vi "funcaoAvaliacaoGoleiroBolaPertoArea.vi"(8 "balls":T1[](array[typedef]), 9 "Robot in":T2, 10 "Estado_Atual":T7(ring), 11 "IA State":T8={"our_robots"=[], "enemy_robots"=[], "balls"=[], "geometry"={"field_length"=0, "field_width"=0, "goal_width"=0, "goal_depth"=0, "center_circle_radius"=0, "defense_width"=0, "defense_depth"=0, "free_kick_from_defense_dist"=0, "penalty_spot_from_field_line_dist"=0, "penalty_line_from_spot_dist"=0, "half_moon_depth"=0, "half_moon_width"=0}, "IA Judge"={"stage"="", "command"="", "our_goalie_id"=0.0, "enemy_goalie_id"=0.0, "command enum"=enum."Halt", "Time"=enum."Azul"}, "Received Timestamp"=timestamp(0 s since 1904-01-01), "Events"={"Touch"=FALSE, "id touch"=0.0, "Ball out of \nVision"=FALSE, "Ball inside \nGoalie area"=FALSE, "Robot not responding"=FALSE, "Robots responding status"=[1.0, 1.0, 1.0, 1.0, 1.0, 1.0], "Enemy Ball \nPossession"=FALSE, "Id ini Possession"=0.0, "Ball Possesion"=FALSE, "Id Possesion"=0.0, "Ball at\nour goal side"=FALSE, "Ball at\ntouchline"=FALSE, "Ball at\nenemy goal side"=FALSE}}) -> (3 "Estado_Novo":T7(ring))   [LabVIEW 2018]
uses:
  2019/VSS/Core/AI Input.ctl
  2019/VSS/Core/AI Robot.ctl
  2019/VSS/Intel/Functions Enum.ctl
  2019/VSS/Intel/AttackerStates.ctl
  2019/VSS/Path Planning/RRT/PathDests.ctl
  2019/VSS/Path Planning/RRT/PathDest.ctl
  2019/VSS/Core/AI Ball.ctl
  2019/VSS/Core/Field Size.ctl
  2019/VSS/Core/AI Judge.ctl
  2019/VSS/Intel/Command Enum.ctl
  2019/VSS/Util/Events/Events.ctl
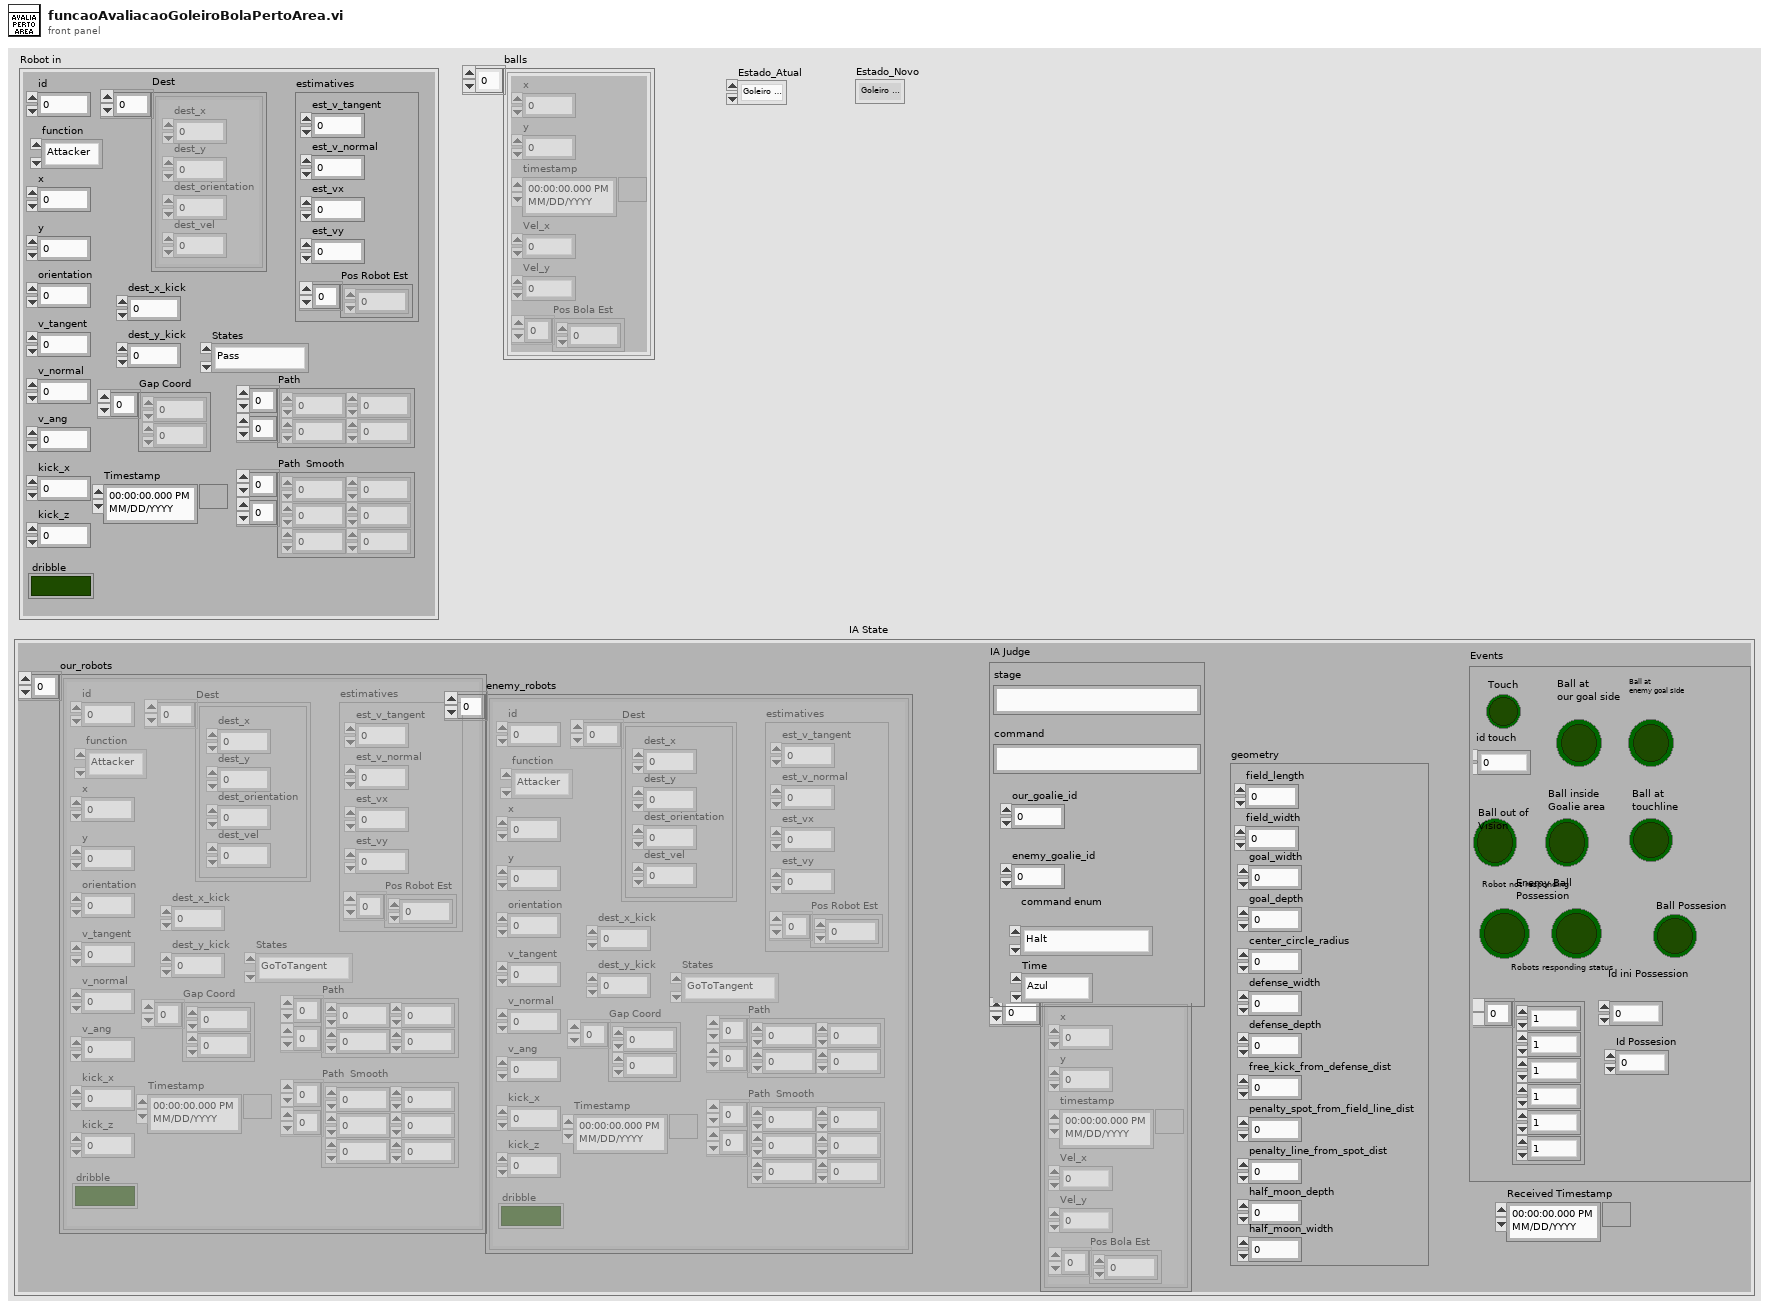
[diagram p1: front panel]
types:
  T1 = typedef "AI Ball.ctl" = cluster{"x":dbl, "y":dbl, "timestamp":timestamp, "Vel_x":dbl, "Vel_y":dbl, "Pos Bola Est":dbl[]}
  T2 = typedef "AI Robot.ctl" = cluster{"id":u32, "function":T3, "x":dbl, "y":dbl, "orientation":dbl, "v_tangent":dbl, "v_normal":dbl, "v_ang":dbl, "kick_x":dbl, "kick_z":dbl, "dribble":bool, "Timestamp":timestamp, "estimatives":cluster{"est_v_tangent":dbl, "est_v_normal":dbl, "est_vx":dbl, "est_vy":dbl, "Pos Robot Est":dbl[]}, "dest_x_kick":dbl, "dest_y_kick":dbl, "Gap Coord":dbl[], "States":T4, "Path ":dbl[][], "Path  Smooth":dbl[][], "Dest":T5}
  T3 = typedef "Functions Enum.ctl" = enum16{"Attacker", "Goalie", "Defender", "Striker", "Goto 0", "Dummy", "Kicker", "ZigZag"}
  T4 = typedef "AttackerStates.ctl" = enum16{"Pass", "GoToTangent", "BallGetting", "GoToKick", "Rotate anti-clockwise", "Rotate Clockwise", ""}
  T5 = typedef "PathDests.ctl" = T6[]
  T6 = typedef "PathDest.ctl" = cluster{"dest_x":dbl, "dest_y":dbl, "dest_orientation":dbl, "dest_vel":dbl}
  T7 = enum16{"Goleiro fora da área", "Alinhar com a bola", "Alinhar com a trave", "Rotacionar", "Aproximar-se da bola", "Posicionar-se na frente da bola"}
  T8 = typedef "AI Input.ctl" = cluster{"our_robots":T2[], "enemy_robots":T2[], "balls":T1[], "geometry":T9, "IA Judge":T10, "Received Timestamp":timestamp, "Events":T12}
  T9 = typedef "Field Size.ctl" = cluster{"field_length":u32, "field_width":u32, "goal_width":u32, "goal_depth":u32, "center_circle_radius":u32, "defense_width":u32, "defense_depth":u32, "free_kick_from_defense_dist":u32, "penalty_spot_from_field_line_dist":u32, "penalty_line_from_spot_dist":u32, "half_moon_depth":u32, "half_moon_width":u32}
  T10 = typedef "AI Judge.ctl" = cluster{"stage":string, "command":string, "our_goalie_id":dbl, "enemy_goalie_id":dbl, "command enum":T11, "Time":enum16{"Azul", "Amarelo"}}
  T11 = typedef "Command Enum.ctl" = enum16{"Halt", "Stop", "Force Start", "PKA Normal Start", "Prepare Kickoff Ally", "PKE Normal Start", "Prepare Kickoff Enemy", "Prepare Penalty Ally", "PPA Normal Start", "Prepare Penalty Enemy", "PPE Normal Start", "Ball Placement Enemy Up", "Ball Placement Enemy Down", "Ball Placement Ally Up", "Ball Placement Ally Mid", "Ball Placement Ally Down", "Indirect Free Enemy", "Indirect Free Ally", "Timeout Enemy", "Timeout Ally", "Goal Enemy", "Goal Ally", "Normal Half Time", "Extra Time Break", "Extra Half Time", "None", "Post Game"}
  T12 = typedef "Events.ctl" = cluster{"Touch":bool, "id touch":dbl, "Ball out of \nVision":bool, "Ball inside \nGoalie area":bool, "Robot not responding":bool, "Robots responding status":dbl[], "Enemy Ball \nPossession":bool, "Id ini Possession":dbl, "Ball Possesion":bool, "Id Possesion":dbl, "Ball at\nour goal side":bool, "Ball at\ntouchline":bool, "Ball at\nenemy goal side":bool}
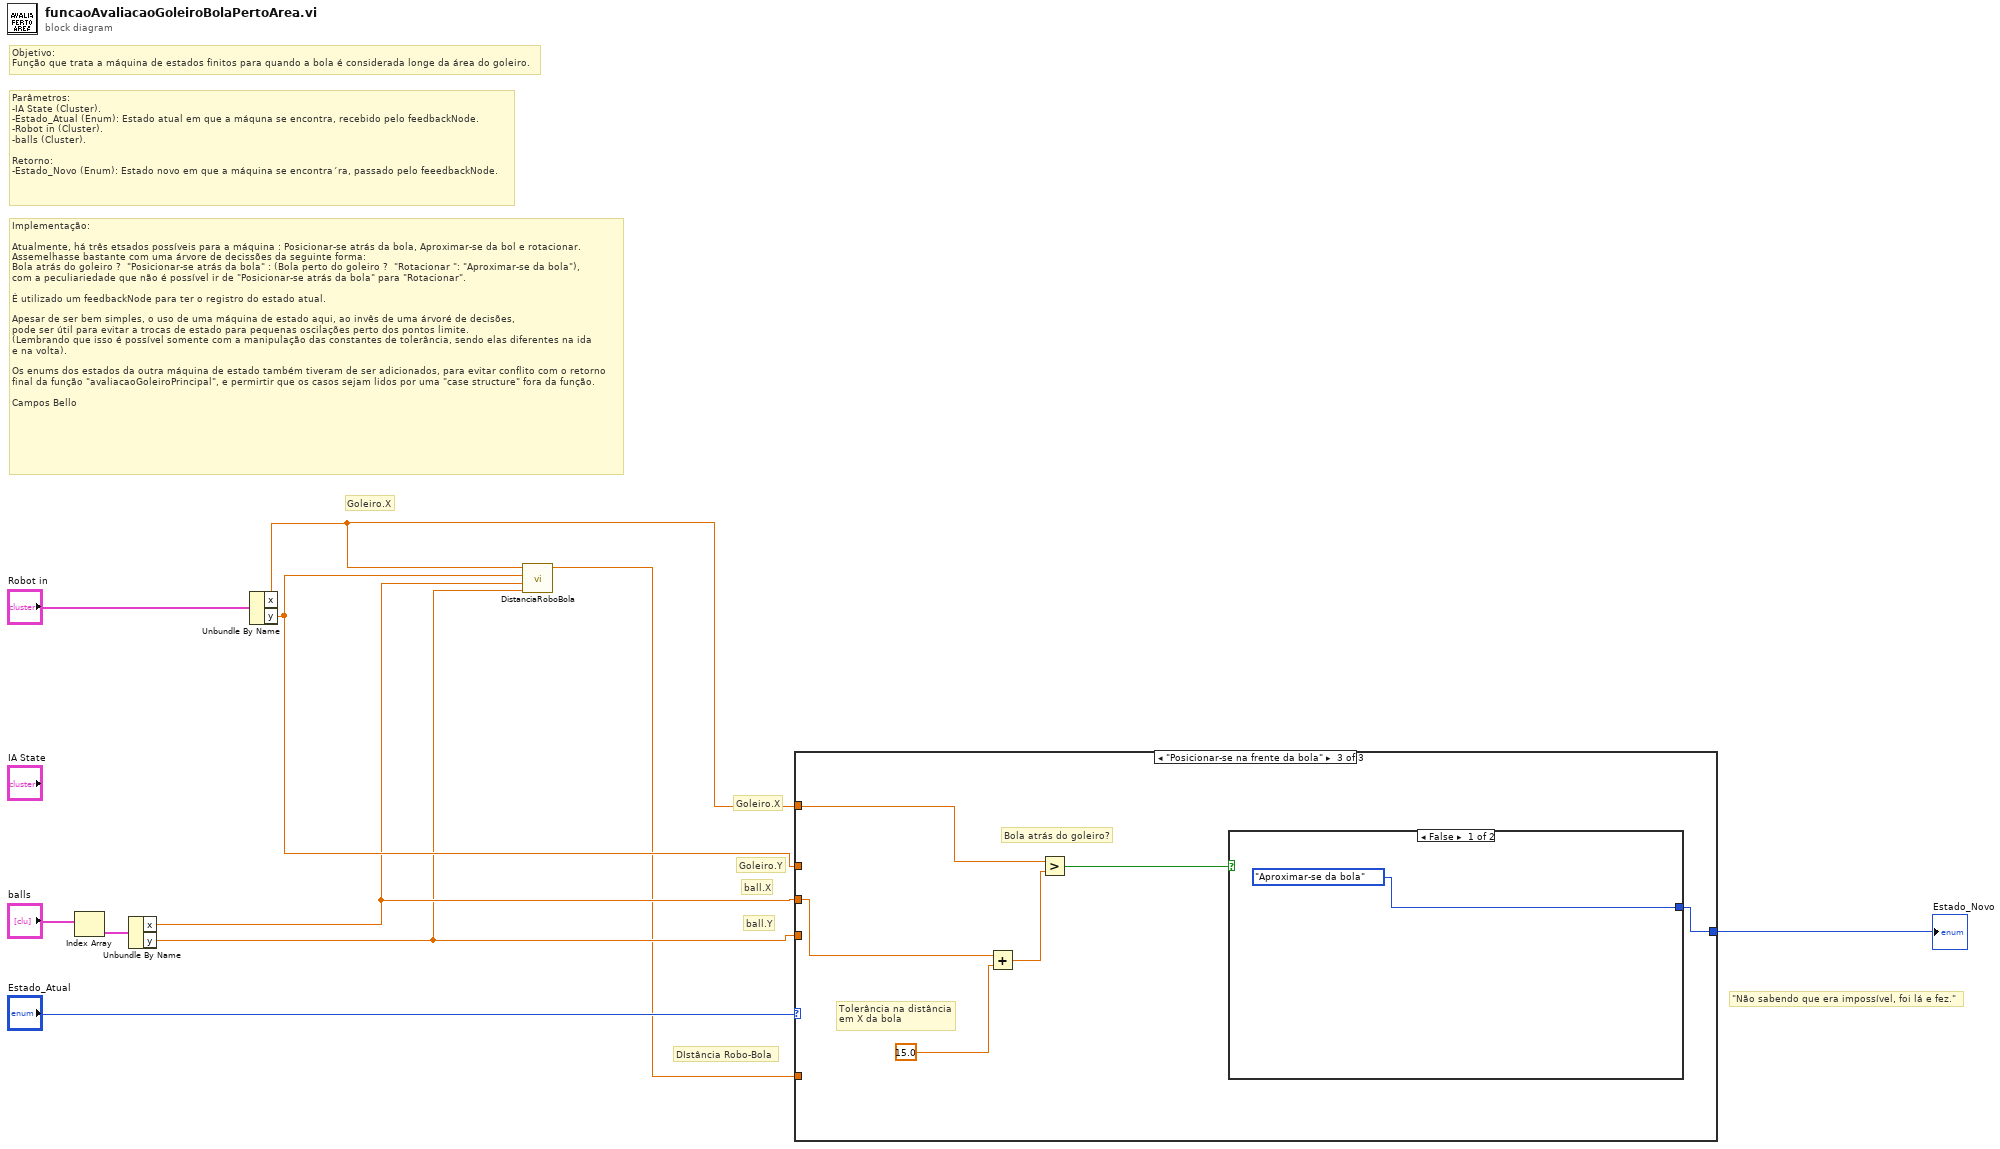
[diagram p0: block diagram]
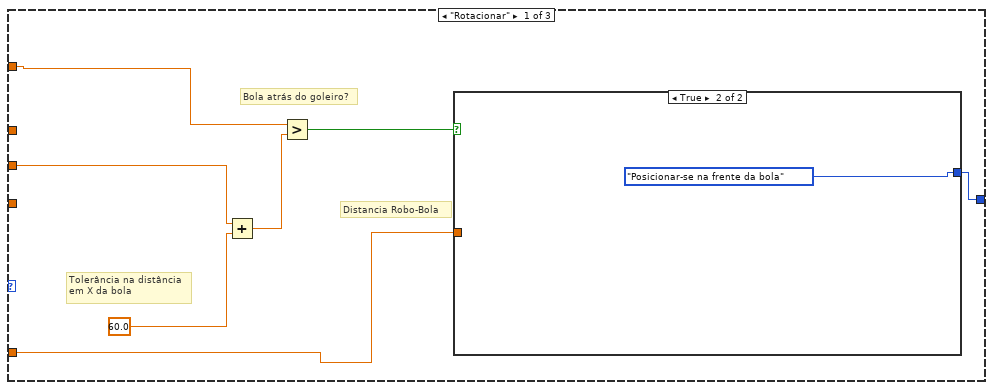
[diagram p2: hidden frame]
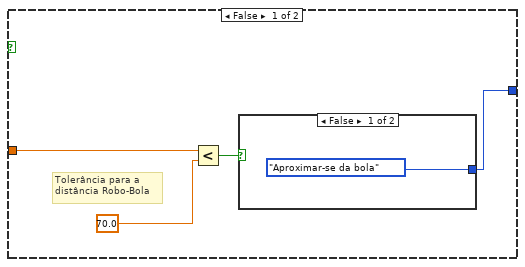
[diagram p3: hidden frame]
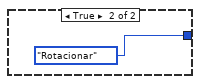
[diagram p4: hidden frame]
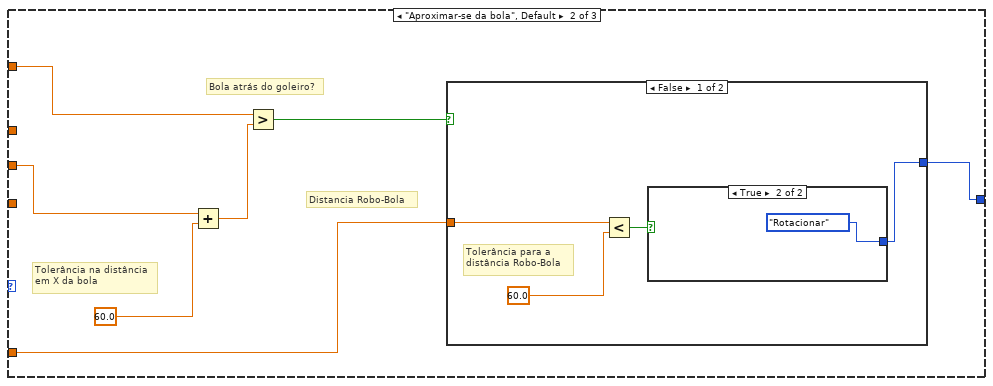
[diagram p5: hidden frame]
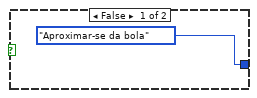
[diagram p6: hidden frame]
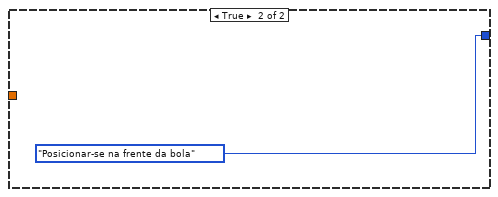
[diagram p7: hidden frame]
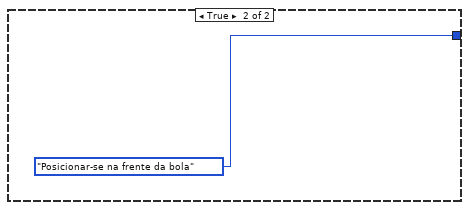
[diagram p8: hidden frame]
diagram:
  # "\"Não sabendo que era impossível, foi lá e fez.\""
  # "Implementação:\n\nAtualmente, há três etsados possíveis para a máquina : Posicionar-se atrás da bola, Aproximar-se da bol e rotacionar.\nAssemelhasse bastante com uma árvore de decissões da seguinte forma: \nBola atrás do goleiro ?  \"Posicionar-se atrás da bola\" : (Bola perto do goleiro ?  \"Rotacionar \": \"Aproximar-se da bola\"), \ncom a peculiariedade que não é possível ir de \"Posicionar-se atrás da bola\" para \"Rotacionar\".\n\nÉ utilizado um feedbackNode para ter o registro do estado atual.\n\nApesar de ser bem simples, o uso de uma máquina de estado aqui, ao invês de uma árvoré de decisões, \npode ser útil para evitar a trocas de estado para pequenas oscilações perto dos pontos limite.\n(Lembrando que isso é possível somente com a manipulação das constantes de tolerância, sendo elas diferentes na ida \ne na volta).\n\nOs enums dos estados da outra máquina de estado também tiveram de ser adicionados, para evitar conflito com o retorno\nfinal da função \"avaliacaoGoleiroPrincipal\", e permirtir que os casos sejam lidos por uma \"case structure\" fora da função.\n\nCampos Bello"
  # "Parâmetros:\n-IA State (Cluster).\n-Estado_Atual (Enum): Estado atual em que a máquna se encontra, recebido pelo feedbackNode.\n-Robot in (Cluster).\n-balls (Cluster).\n\nRetorno:\n-Estado_Novo (Enum): Estado novo em que a máquina se encontra´ra, passado pelo feeedbackNode."
  # "Objetivo:\nFunção que trata a máquina de estados finitos para quando a bola é considerada longe da área do goleiro."
  # "DIstância Robo-Bola"
  # "ball.Y"
  # "ball.X"
  # "Goleiro.Y"
  # "Goleiro.X"
  # "Goleiro.X"
  n1 = Index Array(array="balls") -> (element=w10:T1)  [unwired: 1 in]
  n2 = Unbundle By Name(w10) -> ("x"=w6:dbl, "y"=w5:dbl)
  n3 = Unbundle By Name("Robot in") -> ("x"=w8:dbl, "y"=w7:dbl)
  n4 = call "DistanciaRoboBola.vi"("Y bola"=w5, "X bola"=w6, "Y robo"=w7, "X robo"=w8) -> ("Distância"=w4:dbl)  [unwired: 5 in, 2 out]
  n5 = case shown="\"Posicionar-se na frente da bola\"" "Estado_Atual" {
    tunnel: [w11 w25 w39] -> w3
    tunnel: w8 -> [w14 w29 w41]
    tunnel: w7 -> [_ _ _]
    tunnel: w6 -> [w13 w30 w40]
    tunnel: w5 -> [_ _ _]
    tunnel: w4 -> [w12 w26 _]
    frame "Rotacionar" {
      # "Distancia Robo-Bola"
      # "Bola atrás do goleiro?"
      # "Tolerância na distância\nem X da bola"
      n6 = Add(x=w13, y=60.0) -> (x+y=w16:dbl)
      n7 = Greater?(x=w14, y=w16) -> (0:w15:bool)
      n8 = case shown="True" w15 {
        tunnel: [w18 T7."Posicionar-se na frente da bola" ("Estado_Atual")] -> w11
        tunnel: w12 -> [w21 _]
        frame False {
          # "Tolerância para a \ndistância Robo-Bola"
          n9 = Less?(x=w21, y=70.0) -> (x < y?=w19:bool)
          n10 = case shown="False" w19 {
            tunnel: [T7."Aproximar-se da bola" ("Estado_Atual") T7."Rotacionar" ("Estado_Atual")] -> w18
            frame False {
            }
            frame True {
            }
          }
        }
        frame True {
        }
      }
    }
    frame "Aproximar-se da bola", Default {
      # "Distancia Robo-Bola"
      # "Bola atrás do goleiro?"
      # "Tolerância na distância\nem X da bola"
      n11 = Add(x=w30, y=60.0) -> (x+y=w28:dbl)
      n12 = Greater?(x=w29, y=w28) -> (0:w27:bool)
      n13 = case shown="False" w27 {
        tunnel: [w32 T7."Posicionar-se na frente da bola" ("Estado_Atual")] -> w25
        tunnel: w26 -> [w35 _]
        frame False {
          # "Tolerância para a \ndistância Robo-Bola"
          n14 = Less?(x=w35, y=60.0) -> (x < y?=w33:bool)
          n15 = case shown="True" w33 {
            tunnel: [T7."Aproximar-se da bola" ("Estado_Atual") T7."Rotacionar" ("Estado_Atual")] -> w32
            frame False {
            }
            frame True {
            }
          }
        }
        frame True {
        }
      }
    }
    frame "Posicionar-se na frente da bola" {
      # "Bola atrás do goleiro?"
      # "Tolerância na distância\nem X da bola"
      n16 = Add(x=w40, y=15.0) -> (x+y=w43:dbl)
      n17 = Greater?(x=w41, y=w43) -> (0:w42:bool)
      n18 = case shown="False" w42 {
        tunnel: [T7."Aproximar-se da bola" ("Estado_Atual") T7."Posicionar-se na frente da bola" ("Estado_Atual")] -> w39
        frame False {
        }
        frame True {
        }
      }
    }
  }
  "Estado_Novo" <- w3
